vi "xetIPAddress.vi"(1 "Get/Set":enum16{"Get", "Set"}(ring), 2 "IP Address In":string) -> (0 "IP Address Out":string)   [LabVIEW 2016, in "h.Library.lvlib"]
uses:
  h.Library.lvlib
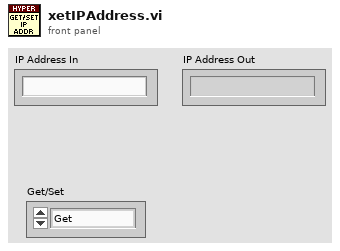
[diagram p1: front panel]
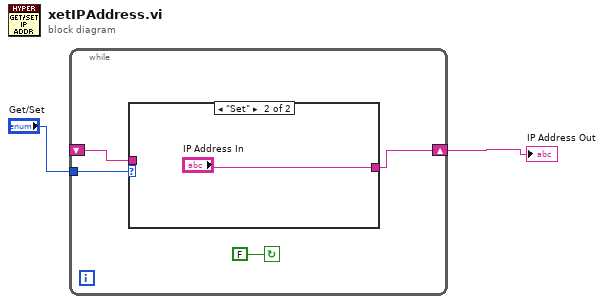
[diagram p0: block diagram]
diagram:
  n1 = while {
    tunnel: "Get/Set" -> [w6]
    shift-right: [w4] -> w1
    shift-left: _ -> [w3]
    stop <- FALSE continue-if-true
    n2 = case shown="\"Set\"" w6 {
      tunnel: [w7 "IP Address In"] -> w4
      tunnel: w3 -> [w7 _]
      frame "Get", Default {
      }
      frame "Set" {
      }
    }
  }
  "IP Address Out" <- w1
